vi "Get software version string.vi"() -> (3 "Software version string":string)   [LabVIEW 2018]
doc: "If unedited, this VI returns either the embedded version number of the EXE it is running inside of (if compiled) or \"LV <main VI verison>.Year.Month.Day\" if running live LabVIEW.\n\nIf this is not desired, then this VI can be modified to either return a fixed string or use any other method desired to look up the version number."
uses:
  <vilib>/Utility/error.llb/Clear Errors.vi
  <userlib>/nLight Error Handling/Log any errors.vi
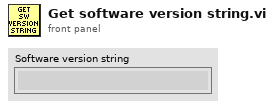
[diagram p1: front panel]
types:
  T1 = cluster{"FileVersion":string, "FileMajorPart":i32, "FileMinorPart":i32, "FileBuildPart":i32, "FilePrivatePart":i32, "Language":string, "LegalCopyright":string, "FileDescription":string, "CompanyName":string, "ProductName":string, "InternalName":string}
  T2 = typedef "LVDateTimeRec.ctl" = cluster{"fractional second":dbl, "second":i32, "minute":i32, "hour":i32, "day of month":i32, "month":i32, "year":i32, "day of week":i32, "day of year":i32, "DST":i32}
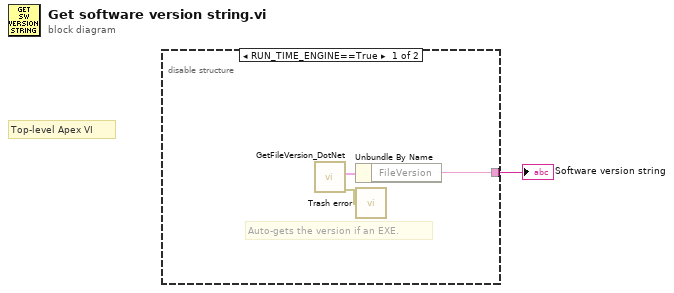
[diagram p0: block diagram]
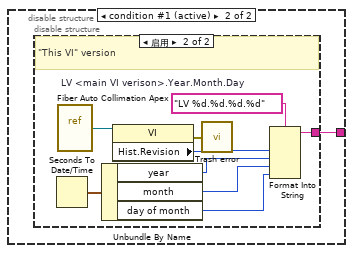
[diagram p2: hidden frame]
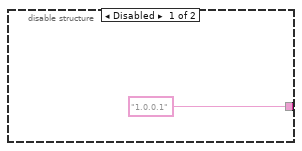
[diagram p3: hidden frame]
diagram:
  # "Top-level Apex VI"
  n1 = disable-structure shown="RUN_TIME_ENGINE==True" {
    disable-tunnel: [w3 w5] -> w1
    frame condition #0 {
      # "Auto-gets the version if an EXE."
      n2 = call <userlib>:"GetFileVersion_DotNet.vi"() -> ("error out"=w2:errorcluster, "File Info Out"=w4:T1)  [unwired: 9 in, 1 out]
      n3 = Unbundle By Name(w4) -> ("FileVersion"=w3:string)
      n4 = call <userlib>:"Trash error.vi"("error in"=w2) -> ()  [unwired: 15 in]
    }
    frame condition #1 (active) {
      n5 = disable-structure shown="启用" {
        disable-tunnel: ["1.0.0.1" w15] -> w5
        frame Disabled {
        }
        frame Enabled {
          w14 = "LV %d.%d.%d.%d"  # LV <main VI verison>.Year.Month.Day
          # "\"This VI\" version"
          n6 = Seconds To Date/Time() -> (date time rec=w12:T2)  [unwired: 2 in]
          n7 = vi-ref "Fiber Auto Collimation Apex.vi"() -> (w8:refnum<vi>)
          n8 = Unbundle By Name(w12) -> ("year"=w11:i32, "month"=w9:i32, "day of month"=w10:i32)
          n9 = property class="VI"(reference=w8) -> (error out=w7:errorcluster, "Hist.Revision"=w13:u32)  [unwired: 1 in, 1 out]
          n10 = call <userlib>:"Trash error.vi"("error in"=w7) -> ()  [unwired: 15 in]
          n11 = Format Into String(format string=w14, w13, w11, w9, w10) -> (resulting string=w15:string)  [unwired: 2 in, 1 out]
        }
      }
    }
  }
  "Software version string" <- w1
